vi "Write Binary Config.vi"(4 "Include Class Name":bool, 6 "byte order (0:big-endian, network order)":T1(ring), 8 "error in (no error)":errorcluster, 11 "Const_DBL in":refnum<class "Const_DBL_1D.lvclass">) -> (0 "error out":errorcluster, 2 "Binary":string, 3 "Const_DBL out":refnum<class "Const_DBL_1D.lvclass">)   [LabVIEW 2021, in "Const_DBL_1D.lvclass"]
uses:
  Const_DBL_1D.lvclass
  Const_DBL_1D.lvclass/Const_DBL_1D.ctl
  Abs_Types/Double Float 1D/Abs_Double Float 1D.lvclass
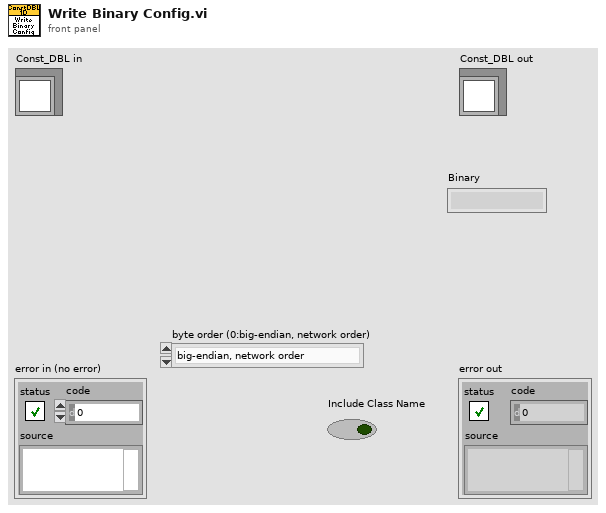
[diagram p1: front panel]
types:
  T1 = enum16{"big-endian, network order", "native, host order", "little-endian"}
  T2 = typedef "Const_DBL_1D.lvclass/Type.ctl" = dbl[]
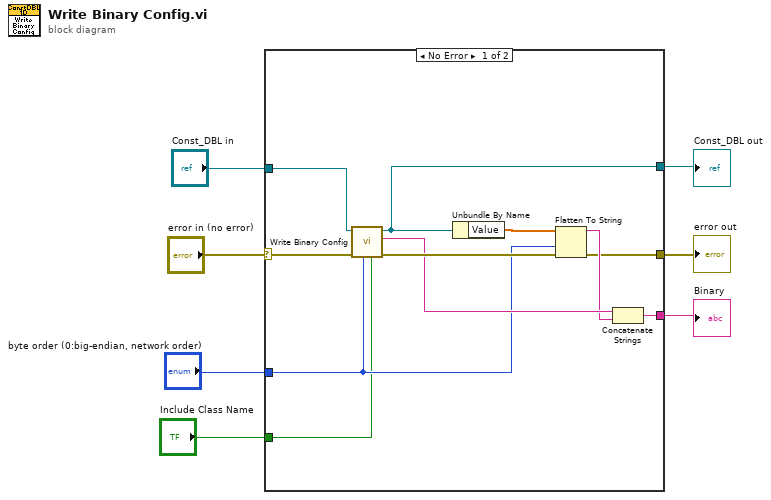
[diagram p0: block diagram]
diagram:
  n1 = case shown="No Error" "error in (no error)" {
    selector: "error in (no error)" -> [w18 w19]
    tunnel: [w9 w19] -> w2
    tunnel: [w16 w20] -> w4
    tunnel: "byte order (0:big-endian, network order)" -> [w11 _]
    tunnel: "Const_DBL in" -> [w17 w20]
    tunnel: [w10 _] -> w3
    tunnel: "Include Class Name" -> [w8 _]
    frame No Error {
      n2 = call-parent "Write Binary Config.vi"("Include Class Name"=w8, "byte order (0:big-endian, network order)"=w11, "error in (no error)"=w18, "Abs_Type in"=w17) -> ("error out"=w14:errorcluster, "Binary"=w13:string, "Abs_Type out"=w16:refnum<class "Const_DBL_1D.lvclass">)  [unwired: 5 in]
      n3 = Unbundle By Name(w16) -> ("Value"=w15:T2)
      n4 = Flatten To String(anything=w15, byte order (0:big-endian, network order)=w11, error in (no error)=w14) -> (data string=w12:string, error out=w9:errorcluster)  [unwired: 1 in, 1 out]
      n5 = Concatenate Strings(w13, w12) -> (w10:string)
    }
    frame Error {
    }
  }
  "error out" <- w2
  "Const_DBL out" <- w4
  "Binary" <- w3
